vi "getEnumSummaryState.vi"(8 "error in (no error)":errorcluster, 10 "valSummaryState":i32, 11 "SalProcess in":refnum<class "SalProcess.lvclass">) -> (0 "error out":errorcluster, 2 "enumSummaryState":T1, 3 "SalProcess out":refnum<class "SalProcess.lvclass">)   [LabVIEW 2018, in "SalProcess.lvclass"]
doc: "Get the enumeration of summary state."
uses:
  SalProcess.lvclass
  TypeDef/summaryState.ctl
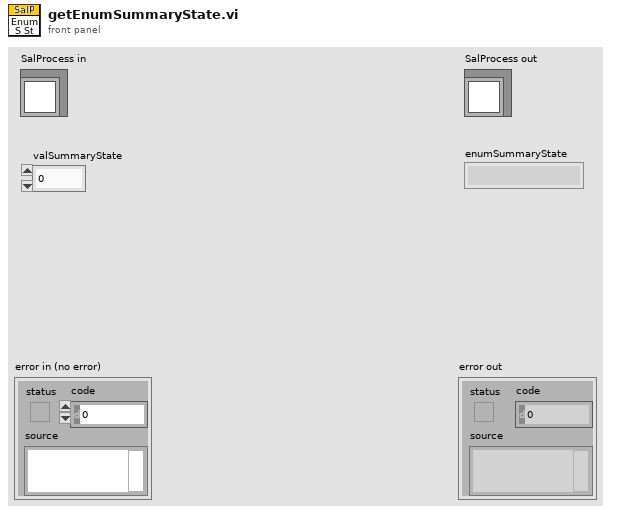
[diagram p1: front panel]
types:
  T1 = typedef "summaryState.ctl" = enum16{"", "DisabledState", "EnabledState", "FaultState", "OfflineState", "StandbyState"}
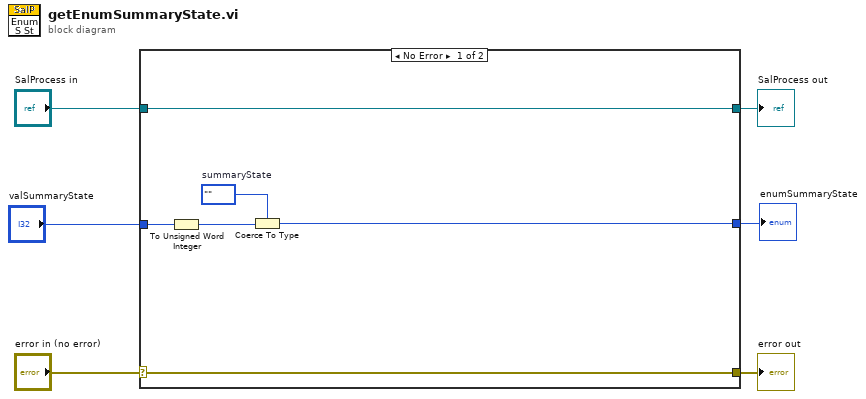
[diagram p0: block diagram]
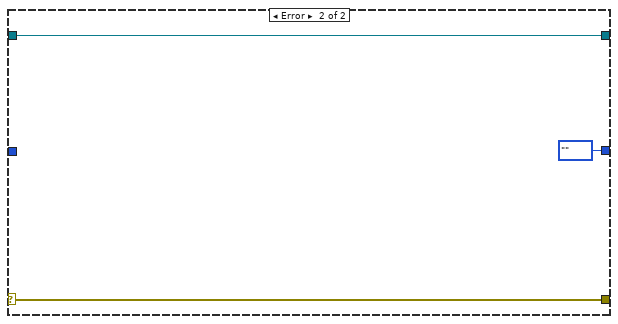
[diagram p2: hidden frame]
diagram:
  n1 = case shown="No Error" "error in (no error)" {
    selector: "error in (no error)" -> [w11 w15]
    tunnel: [w11 w15] -> w5
    tunnel: [w12 w14] -> w3
    tunnel: "SalProcess in" -> [w12 w14]
    tunnel: "valSummaryState" -> [w10 _]
    tunnel: [w7 summaryState."" ("summaryState")] -> w1
    frame No Error {
      w8 = summaryState.""  # summaryState
      n2 = To Unsigned Word Integer(number=w10) -> (unsigned 16bit integer=w9:u16)
      n3 = Coerce To Type(0:w9, 1:w8) -> (2:w7:T1)
    }
    frame Error {
    }
  }
  "error out" <- w5
  "SalProcess out" <- w3
  "enumSummaryState" <- w1
